vi "Periodic Tasks.vi"(8 "error in":errorcluster) -> ()   [LabVIEW 2017]
doc: "This VI runs in parallel to other tasks. It can contain as many user-defined periodic loops as you need. These can carry out PID or other sorts of timed response."
uses:
  <vilib>/Rock Robotics/WPI/ThirdParty/Phoenix-LabVIEW/Motor Controller/Controls/CTRE_Phoenix_MotorControl_ControlMode.ctl
panel:
  in  "Clear":bool
  in  "PIDF":cluster{"P":dbl, "I":dbl, "D":dbl, "F":dbl}
  in  "allowableClosedLoopError":i32=1000
  in  "profileSlotSelect0":i32
  in  "profileSlotSelect1":i32
  out "Motion Profile Status":T1
  in  "Run":bool
  in  "Update Array":bool
  in  "file path (dialog if empty)":path=path "U/UntitledPath (7).txt"
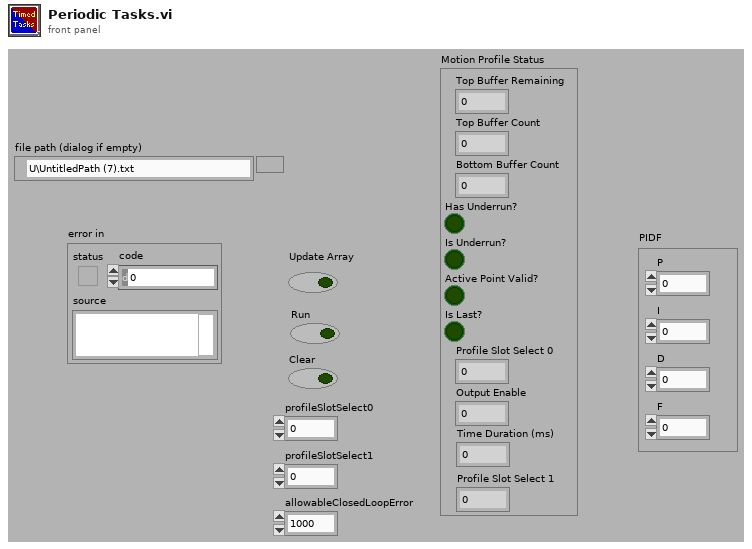
[diagram p1: front panel]
types:
  T1 = cluster{"Top Buffer Remaining":i32, "Top Buffer Count":i32, "Bottom Buffer Count":i32, "Has Underrun?":bool, "Is Underrun?":bool, "Active Point Valid?":bool, "Is Last?":bool, "Profile Slot Select 0":i32, "Output Enable":i32, "Time Duration (ms)":i32, "Profile Slot Select 1":i32}
  T2 = typedef "WPI_MotorControlDeviceRef.ctl" = cluster{"DeviceStatus":errorcluster, "Type":T3, "PWM":cluster{"PWM Channel":T4, "DeadBand":T5}, "CAN":cluster{"Device Number":u8, "SetOutput VI Ref":variant, "GetOutput VI Ref":variant, "Enable VI Ref":variant, "Disable VI Ref":variant, "Data":variant}, "Invert":bool, "DIO PWM":cluster{"PWM \"Enable\" Channel":T4, "DIOChannel":T6, "PWM Rate":dbl}}
  T3 = typedef "WPI_MotorControlType.ctl" = enum16{"PWM", "CAN", "DIO PWM"}
  T4 = typedef "FPGA_DIOPWMChannel.ctl" = enum8{"PWM 0", "PWM 1", "PWM 2", "PWM 3", "PWM 4", "PWM 5", "PWM 6", "PWM 7", "PWM 8", "PWM 9", "PWM MXP 0", "PWM MXP 1", "PWM MXP 2", "PWM MXP 3", "PWM MXP 4", "PWM MXP 5", "PWM MXP 6", "PWM MXP 7", "PWM MXP 8", "PWM MXP 9", "Invalid"}
  T5 = typedef "WPI_PWMDeadband.ctl" = cluster{"Name":string, "maxPositivePwm":i32, "minPositivePwm":i32, "centerPwm":i32, "maxNegativePwm":i32, "minNegativePwm":i32, "angularRange":u16}
  T6 = typedef "FPGA_DIOChannel.ctl" = enum8{"DIO 0", "DIO 1", "DIO 2", "DIO 3", "DIO 4", "DIO 5", "DIO 6", "DIO 7", "DIO 8", "DIO 9", "DIO MXP 0", "DIO MXP 1", "DIO MXP 2", "DIO MXP 3", "DIO MXP 4", "DIO MXP 5", "DIO MXP 6", "DIO MXP 7", "DIO MXP 8", "DIO MXP 9", "DIO MXP 10", "DIO MXP 11", "DIO MXP 12", "DIO MXP 13", "DIO MXP 14", "DIO MXP 15", "SPI Port CS1", "SPI Port CS2", "SPI Port CS3", "SPI Port MISO", "SPI Port MOSI", "Invalid"}
  T7 = typedef "CTRE_Phoenix_MotorControl_ControlMode.ctl" = u16
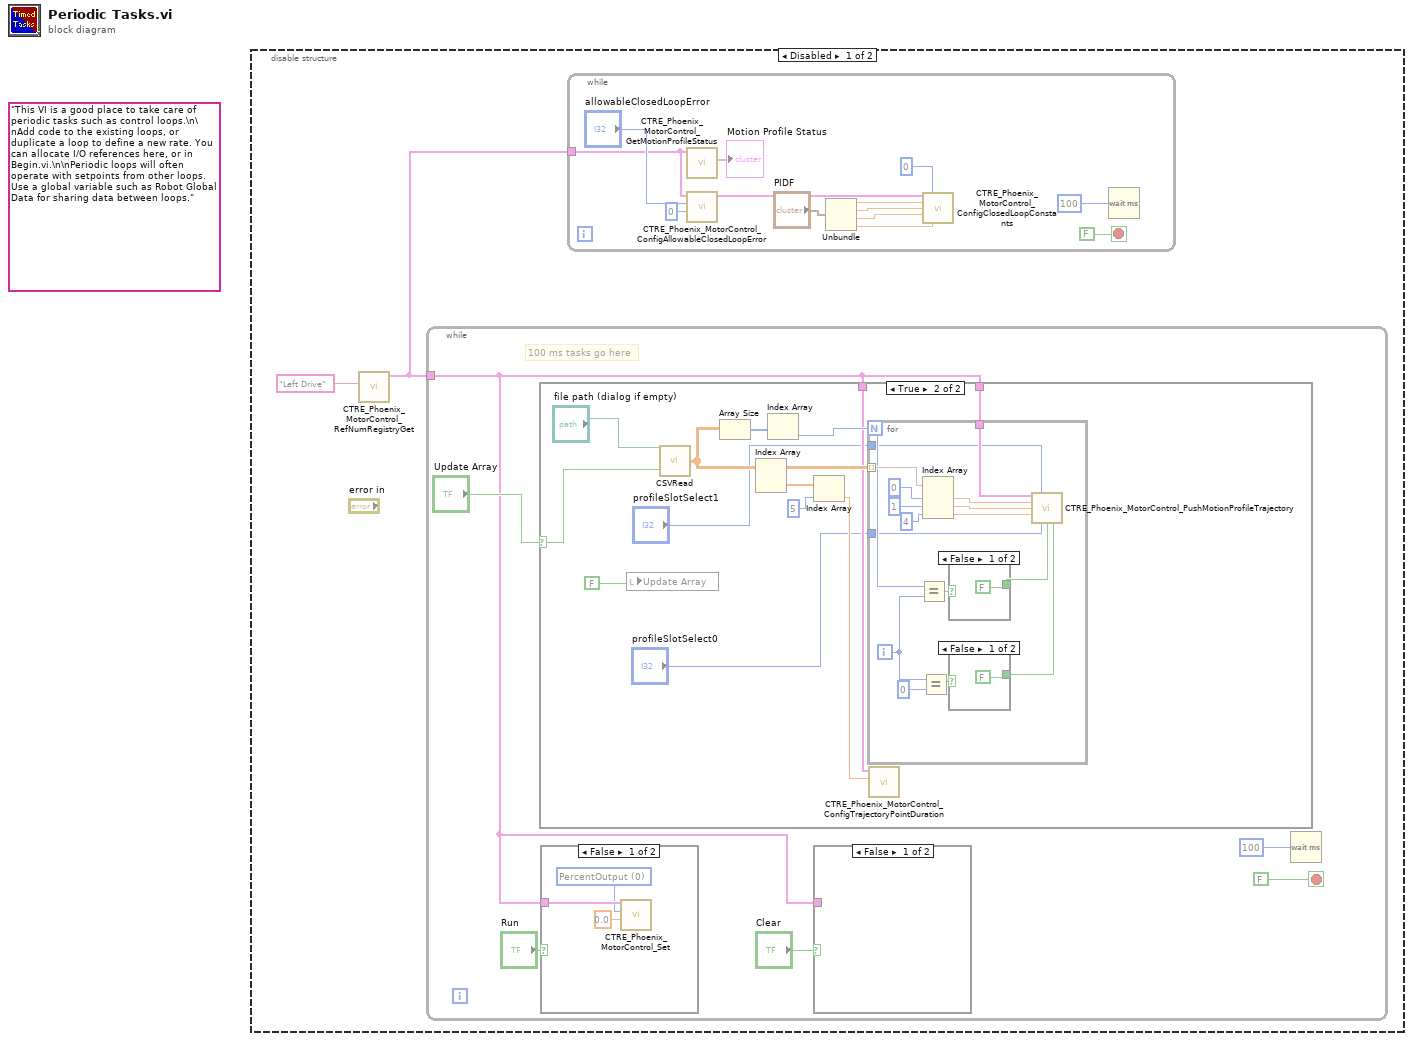
[diagram p0: block diagram]
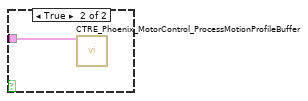
[diagram p2: hidden frame]
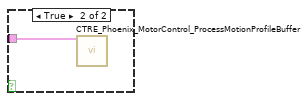
[diagram p3: hidden frame]
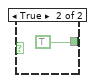
[diagram p5: hidden frame]
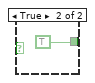
[diagram p6: hidden frame]
diagram:
  (unwired) "This VI is a good place to take care of periodic tasks such as control loops.\n\nAdd code to the existing loops, or duplicate a loop to define a new rate. You can allocate I/O references here, or in Begin.vi.\n\nPeriodic loops will often operate with setpoints from other loops. Use a global variable such as Robot Global Data for sharing data between loops."
  n1 = disable-structure shown="Disabled" {
    frame Disabled {
      n2 = call <vilib>:"CTRE_Phoenix_MotorControl_RefNumRegistryGet.vi"("refnum name"="Left Drive") -> ("PhoenixMotorControlDevRef"=w1:T2)  [unwired: 9 in, 1 out]
      n3 = while {
        tunnel: w1 -> [w16]
        stop <- FALSE stop-if-true
        # "100 ms tasks go here"
        n4 = case shown="True" "Update Array" {
          selector: "Update Array" -> [_ w30]
          tunnel: w16 -> [_ w31]
          tunnel: w16 -> [_ w29]
          frame False {
          }
          frame True {
            n5 = local write "Update Array"(FALSE) -> ()
            n6 = call "CSVRead.vi"("Update Array"=w30, "file path (dialog if empty) 2"="file path (dialog if empty)") -> ("all rows 2"=w36:dbl[][])
            n7 = Array Size(array=w36) -> (size(s)=w38:i32[])
            n8 = Index Array(array=w36) -> (element=w35:dbl[])  [unwired: 2 in]
            n9 = Index Array(array=w38) -> (element=w37:i32)  [unwired: 1 in]
            n10 = Index Array(array=w35, index=5) -> (element=w34:dbl)
            n11 = for {
              N: w37 -> [w50]
              tunnel: w36 -> [w56] mode=indexing
              tunnel: w31 -> [w51]
              tunnel: "profileSlotSelect0" -> [w43]
              tunnel: "profileSlotSelect1" -> [w42]
              i -> [w48]
              n12 = Equal?(x=w50, y=w48) -> (x = y?=w45:bool)
              n13 = Equal?(x=w48, y=0) -> (x = y?=w46:bool)
              n14 = Index Array(array=w56, index #1=0 ("index"), index #2=1 ("index"), index #3=4 ("index")) -> (element #1=w54:dbl, element #2=w53:dbl, element #3=w52:dbl)
              n15 = case shown="False" w45 {
                tunnel: [FALSE TRUE] -> w49
                frame False {
                }
                frame True {
                }
              }
              n16 = case shown="False" w46 {
                tunnel: [FALSE TRUE] -> w44
                frame False {
                }
                frame True {
                }
              }
              n17 = call <vilib>:"CTRE_Phoenix_MotorControl_PushMotionProfileTrajectory.vi"("PhoenixMotorControlDevRef"=w51, "profileSlotSelect1"=w42, "position"=w54, "velocity"=w53, "auxiliaryPos"=w52, "profileSlotSelect0"=w43, "isLastPoint?"=w49, "Zero Position?"=w44) -> ()  [unwired: 6 in, 2 out]
            }
            n18 = call <vilib>:"CTRE_Phoenix_MotorControl_ConfigTrajectoryPointDuration.vi"("durationMs"=w34, "PhoenixMotorControlDevRef"=w29) -> ()  [unwired: 8 in, 2 out]
          }
        }
        n19 = case shown="False" "Run" {
          tunnel: w16 -> [w25 w26]
          frame False {
            w24 = T7 0 items=["PercentOutput"=0, "Position"=1, "Velocity"=2, "Current"=3, "Follower"=5, "MotionProfile"=6, "MotionMagic"=7, "MotionMagicArc"=8, "MotionProfileArc"=10, "Disabled"=15] ("Control Mode")
            n20 = call "CTRE_Phoenix_MotorControl_Set.vi"("Output"=0.0, "Control Mode"=w24, "PhoenixMotorControlDevRef"=w25) -> ()  [unwired: 7 in, 2 out]
          }
          frame True {
            n21 = call <vilib>:"CTRE_Phoenix_MotorControl_ProcessMotionProfileBuffer.vi"("PhoenixMotorControlDevRef"=w26) -> ()  [unwired: 13 in, 2 out]
          }
        }
        n22 = case shown="False" "Clear" {
          tunnel: w16 -> [_ w22]
          frame False {
          }
          frame True {
            n23 = call <vilib>:"CTRE_Phoenix_MotorControl_ProcessMotionProfileBuffer.vi"("PhoenixMotorControlDevRef"=w22) -> ()  [unwired: 13 in, 2 out]
          }
        }
        n24 = Wait (ms)(milliseconds to wait=u32 100) -> ()  [unwired: 1 out]
      }
      n25 = while {
        tunnel: w1 -> [w3]
        stop <- FALSE stop-if-true
        n26 = call <vilib>:"CTRE_Phoenix_MotorControl_GetMotionProfileStatus.vi"("PhoenixMotorControlDevRef"=w3) -> ("Motion Profile Status"=→"Motion Profile Status":T1)  [unwired: 8 in, 2 out]
        n27 = call <vilib>:"CTRE_Phoenix_MotorControl_ConfigAllowableClosedLoopError.vi"("slotIdx"=u32 0, "allowableClosedLoopError"="allowableClosedLoopError", "PhoenixMotorControlDevRef"=w3) -> ("PhoenixMotorControlDevRef"=w10:T2)  [unwired: 7 in, 1 out]
        n28 = Unbundle("PIDF") -> ("P"=w8:dbl, "I"=w7:dbl, "D"=w6:dbl, "F"=w5:dbl)
        n29 = call <vilib>:"CTRE_Phoenix_MotorControl_ConfigClosedLoopConstants.vi"("PhoenixMotorControlDevRef"=w10, "slotIdx"=0, "P"=w8, "I"=w7, "D"=w6, "F"=w5) -> ()  [unwired: 8 in, 2 out]
        n30 = Wait (ms)(milliseconds to wait=u32 100) -> ()  [unwired: 1 out]
      }
    }
    frame Enabled {
    }
  }
